vi "Init.vi"(8 "error in":errorcluster, 11 "ControllerBase in":refnum<class "ControllerBase.lvclass">) -> (0 "error out":errorcluster, 3 "ControllerBase out":refnum<class "ControllerBase.lvclass">)   [LabVIEW 2025, in "ControllerBase.lvclass"]
uses:
  ControllerBase.lvclass
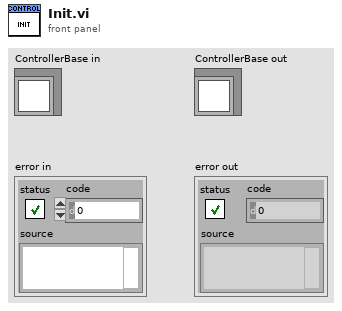
[diagram p1: front panel]
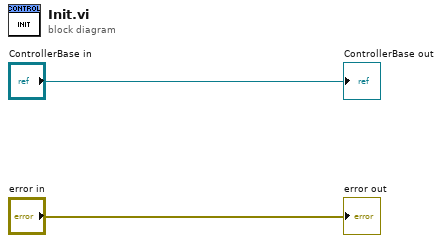
[diagram p0: block diagram]
diagram:
  "error out" <- "error in"
  "ControllerBase out" <- "ControllerBase in"
